vi "a.vi"() -> ()   [LabVIEW 2017]
panel:
  out "前面板窗口:状态":T1(ring)
  in  "打开":bool
  in  "a":dbl
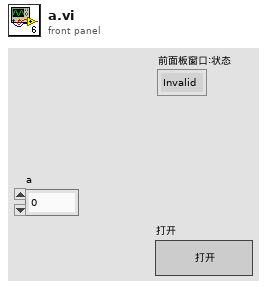
[diagram p1: front panel]
types:
  T1 = enum32{"Invalid", "Standard", "Closed", "Hidden", "Minimized", "Maximized"}
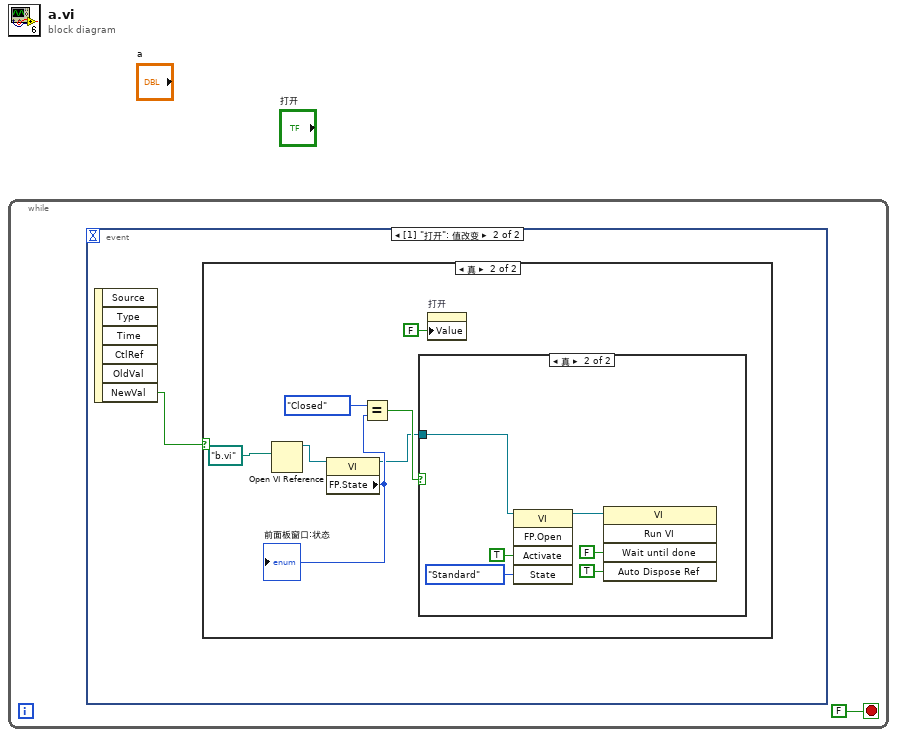
[diagram p0: block diagram]
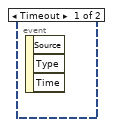
[diagram p2: hidden frame]
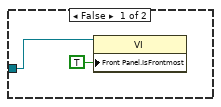
[diagram p4: hidden frame]
diagram:
  n1 = while {
    stop <- FALSE stop-if-true
    n2 = event shown="[1] \"打开\": 值改变" {
      selector: _ -> [_ _]
      dyn-events: _ -> [_ _]
      timeout: _ -> [_ _]
      event Timeout {
        n3 = event-data() -> ()  [unwired: 1 in, 3 out]
      }
      event "打开": Value Change {
        n4 = event-data() -> ("NewVal"=w2:bool)  [unwired: 1 in, 5 out]
        n5 = case shown="真" w2 {
          frame False {
          }
          frame True {
            n6 = Open VI Reference(vi path=path "b.vi") -> (vi reference=w8:refnum<vi>)  [unwired: 5 in, 1 out]
            n7 = property class="VI"(reference=w8) -> (reference out=w4:refnum<vi>, "FP.State"=w7:T1)  [unwired: 1 in, 1 out]
            "前面板窗口:状态" <- w7
            n8 = Equal?(x=T1."Closed", y=w7) -> (x = y?=w5:bool)
            n9 = case shown="真" w5 {
              tunnel: w4 -> [w10 w12]
              frame False {
                n10 = property class="VI"(reference=w10, "Front Panel.IsFrontmost"=TRUE ("前面板窗口:在最前")) -> ()  [unwired: 1 in, 2 out]
              }
              frame True {
                n11 = invoke class="VI" method="FP.Open"(reference=w12, "Activate"=TRUE ("激活？"), "State"=T1."Standard" ("状态")) -> (reference out=w15:refnum<vi>)  [unwired: 2 in, 4 out]
                n12 = invoke class="VI" method="Run VI"(reference=w15, "Wait until done"=FALSE ("结束前等待"), "Auto Dispose Ref"=TRUE ("自动销毁引用")) -> ()  [unwired: 2 in, 5 out]
              }
            }
            n13 = property on="打开" class="Bool (严格)"("Value"=FALSE ("打开")) -> ()  [unwired: 2 in, 2 out]
          }
        }
      }
    }
  }
